vi "AlliGator Overlay Decay Fit Parameter Map in Original Image.vi"(5 "Decay Fit Parameter Map Color Scale Refnum":refnum<vi>, 7 "Image Color Scale Refnum":refnum<vi>, 8 "Error In":errorcluster, 10 "Destination Image Control Refnum":T1 caption="Source Image Refnum", 11 "AlliGator IV DVR in":refnum<data-value>) -> (0 "Error Out":errorcluster, 1 "# Overlay Pixels":i32, 3 "AlliGator IV DVR out":refnum<data-value>)   [LabVIEW 2021, in "AlliGator Decay Fit Parameter Map.lvlib"]
doc: "Overlays the Decay Fit Parameter Map on the Source Image."
uses:
  AlliGator Decay Fit Parameter Map.lvlib
  Image/Image Control Refnum.ctl
  Internal Variables/AlliGator Internal Variables v2.ctl
  <vilib>/vision/Image Controls.llb/IMAQ Image.ctl
  Internal Variables/AlliGator Gate Image Set.ctl
  Files/AlliGator FLI Dataset Type.ctl
  Files/AlliGator Data Series Type.ctl
  Dual-Channel Datasets/AlliGator Dataset Channel.ctl
  Settings/AlliGator Gate Arithmetic.ctl
  Source Image/AlliGator Displayed Image.ctl
  Image/Named ROI Description.ctl
  Phasor Graph/AlliGator Decay Metadata v3.ctl
  Decay Analysis/Decay Preprocessing/AlliGator Decay Background Subtraction Info.ctl
  Decay Analysis/Decay Preprocessing/AlliGator Baseline Subtraction Method.ctl
  Graphs/XY Graph/XY Graph Plot Shift Parameters.ctl
  Graphs/XY Graph/XY Graph Plot Shift Method.ctl
  Decay Analysis/Decay Preprocessing/AlliGator Decay Extrapolation Parameters.ctl
  Phasor/Calibration Phasor (m, phi).ctl
  Phasor/Phasor Reference Series.ctl
  Phasor/Phasor Calibration Map v2.ctl
  Phasor/Phasor (g, s).ctl
  Phasor Graph/AlliGator Raw Phasor Plot Data v4.ctl
  Phasor/Phasor Standard Deviation Options.ctl
  Phasor Plot/AlliGator Phasor Multi-Harmonic Data.ctl
  Phasor/Phasor Harmonic Data.ctl
  AlliGator Decay Fit Options & Parameters v2.ctl
  Fits/IRF(X)PSED/Decay Fit Options v2.ctl
  Fits/Decay Convolution/Decay Model.ctl
  Fits/Residual Type.ctl
  Fits/IRF(X)PSED/Fit Weights Type.ctl
  Fits/Non-linear Fitting Method v2.ctl
  Fits/Fit Calculation Method.ctl
  Fits/Non-linear Fitting Algorithm.ctl
  Decay Analysis/Decay Fit/AlliGator Decay Fit Parameter Constraints 2.ctl
  Fits/IRF(X)PSED/Decay Fit Parameters In List.ctl
  Fits/IRF(X)PSED/MLE Baseline Offset Type.ctl
  Decay Analysis/Decay Preprocessing/AlliGator Decay Preprocessing Parameters.ctl
  Fits/IRF(X)PSED/Decay Fit Parameters & Derived Quantities List v2.ctl
  AlliGator Parameter Maps Data.ctl
  Settings/AlliGator Settings List.ctl
  Palette/Limit+NaN Colors.ctl
  Globals, Variables, Constants/AlliGator Variables List.ctl
  Palette/Image Palette Information.ctl
  Image/Image Display Palette Type.ctl
  Variant/Variant to Data/Variant to Boolean.vi
  Error/Error.lvlib
  Image/Image.lvlib
  Settings/AlliGator Settings.lvlib
  Variant/Variant to Data/Variant to Data.lvlib
  <vilib>/vision/NI_Vision_Development_Module.lvlib
  Time/Time.lvlib
  Globals, Variables, Constants/AlliGator Globals, Variables & Constants.lvlib
  Palette/Palette.lvlib
  Utilities/Utilities.lvlib
  Phasor/Phasor.lvlib
  Decay Analysis/Decay Preprocessing/AlliGator Decay Preprocessing.lvlib
  Graphs/XY Graph/XY Graph Add-Ons.lvlib
  Phasor Graph/AlliGator Phasor Graph.lvlib
  Files/AlliGator Files.lvlib
  Phasor Plot/AlliGator Phasor Plot.lvlib
  Source Image/AlliGator Source Image.lvlib
  Internal Variables/AlliGator Internal Variables.lvlib
  Fits/Fits.lvlib
  Decay Analysis/Decay Fit/AlliGator Decay Fit.lvlib
  Dual-Channel Datasets/AlliGator Dual-Channel Datasets.lvlib
panel:
  out "Overlay Copy (s)":dbl
  out "Overlay Erase (s)":dbl
  out "Overlay Compute (s)":dbl
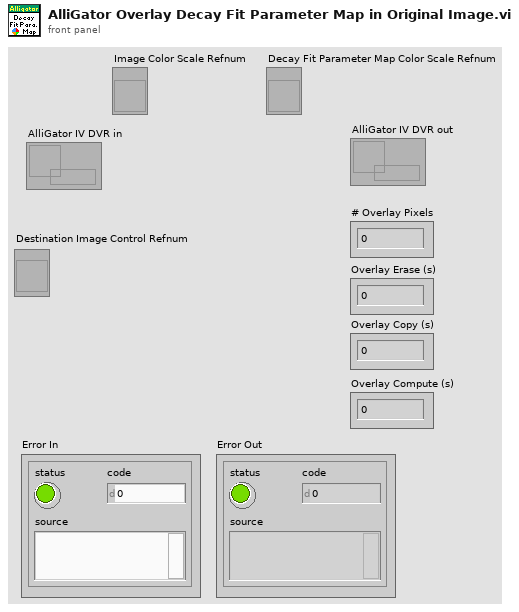
[diagram p1: front panel]
types:
  T1 = typedef "Image.lvlib/Image Control Refnum.ctl" = refnum<vi>
  T2 = typedef "Palette.lvlib/Limit+NaN Colors.ctl" = cluster{"Color Scale High Color":cluster{"Red (or Hue) value":u8, "Green (or Sat) value":u8, "Blue (or Light or Val) value":u8}, "Color Scale Low Color":cluster{"Red (or Hue) value":u8, "Green (or Sat) value":u8, "Blue (or Light or Val) value":u8}, "NaN Color":cluster{"Red (or Hue) value":u8, "Green (or Sat) value":u8, "Blue (or Light or Val) value":u8}}
  T3 = typedef "AlliGator Settings.lvlib/AlliGator Settings List.ctl" = enum16{"GUI:Visible Settings Tab", "GUI:Last Run Version", "Source Image:Use Image Histogram for Contrast", "Source Image:Low Count Pixels Rejection Options", "Source Image:High Count Pixels Rejection Options", "Source Image:Use Image Brightness", "Source Image:Blend Overlay with Image Background", "Source Image:Use Fixed ROI Diameter", "Source Image:ROI Diameter", "Source Image:ROI Center Color", "Source Image:Peak Threshold", "Source Image:Intensity Threshold", "Source Image:Image Binning Options", "Source Image:Image Smoothing Options", "Source Image:Image Histogram Active", "Source Image:Invert Binary Mask", "Source Image:Hot Pixel Removal", "Source Image:Overlay Analyzed ROI Center", "Source Image:Auto-Adjust Contrast", "Source Image:Histogram Lower Percentile", "Source Image:Histogram Upper Percentile", "Source Image:Save Source Image", "Source Image:Scale Bar Options", "Source Image:Image Resolution (Pixel Size)", "Source Image:Flatfield Correction", "Source Image:Show Dead Left Columns Correction", "Source Image:Dead Left Columns Correction", "Source Image:Image Pre-Processing Operations Order", "Source Image:Overlay ROI Median", "Source Image:Median Overlay Color", "Data Information:Gate Width", "Data Information:Nanotime Gate Separation", "Data Information:Macrotime Gate Separation", "Data Information:Gate Step", "Data Information:# Gates", "Data Information:Gate Image Exposure", "Data Information:Gate Image Integration", "Data Information:Gates to Skip", "Data Information:Gates to Keep", "Data Information:Define Gates to", "Data Information:Channel Name", "Data Information:Available Channel Names", "Data Information:Channel Arithmetic", "Data Information:Background File Subtraction", "Data Information:Background File", "Data Information:Background Scaling Factor", "Data Information:Background Pile-up Correction", "Data Information:Background Pixel Well Capacity", "Data Information:Laser Period", "Data Information:SYNC Period", "Data Information:Pile-up Correction", "Data Information:Pixel Well Capacity", "Data Information:Dataset Scaling Factor", "Fluorescence Decay_Decay Pre-Processing:Reverse Gates", "Fluorescence Decay_Decay Pre-Processing:Verbose Decay Pre-Processing", "Fluorescence Decay_Decay Pre-Processing:Use Decay Pre-Processing", "Fluorescence Decay_Decay Pre-Processing:Background Subtraction", "Fluorescence Decay_Decay Pre-Processing:Background Definition Range", "Fluorescence Decay_Decay Pre-Processing:Baseline Subtraction Method", "Fluorescence Decay_Decay Pre-Processing:Decay Pre-Processing Operations Order", "Fluorescence Decay_Decay Pre-Processing:Smoothing Parameter", "Fluorescence Decay_Decay Pre-Processing:Shift Decay", "Fluorescence Decay_Decay Pre-Processing:Decay Shift Parameters", "Fluorescence Decay_Decay Pre-Processing:Fold Decay", "Fluorescence Decay_Decay Pre-Processing:# Folds", "Fluorescence Decay_Decay Pre-Processing:1-Normalize Decay", "Fluorescence Decay_Decay Pre-Processing:[0-1]-Normalize Decay", "Fluorescence Decay_Decay Pre-Processing:Smoothen Decay", "Fluorescence Decay_Decay Pre-Processing:Extrapolate Decay", "Fluorescence Decay_Decay Pre-Processing:Use Periodicity", "Fluorescence Decay_Decay Pre-Processing:Use Cursors", "Fluorescence Decay_Decay Pre-Processing:Tail Fraction", "Fluorescence Decay_Decay Pre-Processing:Head Fraction", "Fluorescence Decay_Decay Pre-Processing:Additional Points", "Fluorescence Decay_Decay Pre-Processing:Straighten Decay", "Fluorescence Decay_Decay Pre-Processing:Constant Background", "Fluorescence Decay_Decay Pre-Processing:Pixel-Normalize Decay", "Fluorescence Decay_Advanced Analysis:Extract IRF instead of Decay", "Fluorescence Decay_Advanced Analysis:IRF Extraction Options", "Fluorescence Decay_Advanced Analysis:IRF Optimization Options", "Fluorescence Decay_Advanced Analysis:Square Pulse Options", "Fluorescence Decay_Advanced Analysis:IRF Order", "Fluorescence Decay_Advanced Analysis:IRF Time Constants", "Fluorescence Decay_Advanced Analysis:Wavelet Analysis Options", "Fluorescence Decay_Advanced Analysis:Average Lifetime Options", "Fluorescence Decay_Fit Options:Fit Options", "Fluorescence Decay_Fit Options:Use Legacy Fitting Approach", "Fluorescence Decay_Fit Options:Use Data Information Laser Period", "Fluorescence Decay_Fit Parameters:Displayed Fit Parameters", "Fluorescence Decay_Fit Parameters:Fit Parameter Constraints", "Fluorescence Decay_Fit Parameters:Export Tabulated Results", "Fluorescence Decay_Fit Parameters:MLE Baseline Offset Type", "Fluorescence Decay_Fit Parameters:MLE Baseline Offset", "Fluorescence Decay_Fit Parameters:Guess Parameter Names", "Fluorescence Decay_Fit Parameters:Guess Parameter Values", "Fluorescence Decay_Fit Parameters:Guess Parameters Options", "Fluorescence Decay_Fit Parameters:Optimal Offset Selection Criterion", "Fluorescence Decay_Styles:Show Last Decay Only", "Fluorescence Decay_Styles:Decay Graph Color Array", "Fluorescence Decay:Decay Graph Active", "Fluorescence Decay Statistics:Min Peak Value", "Fluorescence Decay Statistics:Reject Low Decay Peak Pixels", "Fluorescence Decay Statistics:Reject High Decay Peak Pixels", "Fluorescence Decay Statistics:Max Peak Value", "Time Traces:Use File Timestamp", "Time Traces:Time Step", "Time Traces:Use Intensity Correction File", "Time Traces:Intensity Correction File", "Phasor Plot:Phasor Plot Smoothing Options", "Phasor Plot:Phasor Plot Size", "Phasor Plot:Phasor Plot Graphics Options", "Phasor Plot:Cumulative Phasor Plot", "Phasor Plot:Use Phasor Brightness", "Phasor Plot:Blend Overlay with Phasor Background", "Phasor Plot:Save Phasor Plot", "Phasor Plot:Show References", "Phasor Plot:Phasor Ratio Decay Range", "Phasor Plot:Exponential Fading", "Phasor Plot:Phasor Ratio Reference Colors", "Phasor Plot:Reference Radius", "Phasor Plot:Show Color Map Vertices", "Phasor Plot:Phasor Plot Active", "Phasor Plot:Phasor Ratio Color Map Type", "Phasor Plot:Phasor Ratio Color Map", "Phasor Plot:Phasor Ratio Display Range", "Phasor Plot:Selected Image ROI(s)", "Phasor Plot:All Image ROIs", "Phasor Plot:Selected Phasor Plot ROI(s)", "Phasor Plot:All Phasor Plot ROIs", "Phasor Plot:Phasor Ratio Color-Coded Quantity", "Phasor Plot:Store Phasor Harmonics", "Phasor Plot:Draw Reference Segment", "Phasor Plot:User-Defined Quantity", "Phasor Plot:Color Scale High Color", "Phasor Plot:Color Scale Low Color", "Phasor Graph:Phasor Frequency", "Phasor Graph:Phasor Ratio Type", "Phasor Graph:Pixel-level Phasor Computation", "Phasor Graph:Save Phasor Graph", "Phasor Graph:Phasor Graph Active", "Phasor Graph:Phasor SDV Options", "Phasor Calibration:Use Backup Calibration if needed", "Phasor Graph:Define Shortest Lifetime as", "Phasor Calibration:Backup Calibration Type", "Phasor Calibration:Calibration Type", "Phasor Calibration:Calibration Lifetime", "Phasor Calibration:Calibration Map Algorithm", "Single-Exponential Phasor Locus (SEPL):Gate Parameters", "Single-Exponential Phasor Locus (SEPL):User-defined Gate", "Single-Exponential Phasor Locus (SEPL):User-defined IRF", "Single-Exponential Phasor Locus (SEPL):Phasor Parameters", "Single-Exponential Phasor Locus (SEPL):Decay & IRF Parameters", "Single-Exponential Phasor Locus (SEPL):Display Parameters", "Lifetime Analysis:Decay Analysis Parameters", "Lifetime Analysis:Lifetime Map Active", "Plugins:Python Settings", "Miscellaneous:Verbose Mode", "Miscellaneous:Beep after Script", "Miscellaneous:Saved Image File Format", "Miscellaneous:Exported Gate Image Settings", "Miscellaneous:Include Loading in Timing", "Miscellaneous:Verbose Settings Mode", "Miscellaneous:Histogram Options", "Miscellaneous:Beep on Error", "Miscellaneous:# Logical Processors Used", "Miscellaneous:ROI Description Max Characters", "Miscellaneous:Verbose Error Mode", "Miscellaneous:Transparent Mask Color"}
  T4 = cluster{"Red (or Hue) value":u8, "Green (or Sat) value":u8, "Blue (or Light or Val) value":u8}
  T5 = typedef "IMAQ Image.ctl" = refnum<image>
  T6 = typedef "AlliGator Globals, Variables & Constants.lvlib/AlliGator Variables List.ctl" = enum16{"---- GUI ----", "GUI:Initialization Status", "GUI:State Indicators Refnum", "GUI:Original AlliGator Menu Items", "GUI:Current Action Loop State", "GUI:Script in progress", "GUI:Playback", "GUI:Loop Playback", "GUI:Search ROI Used", "GUI:Search ROI", "Decay Graph Max Legend Size", "Intensity Graph Max Legend Size", "Decay Statistics Graph Max Legend Size", "Phasor Graph Max Legend Size", "Phasor Ratio Graph Max Legend Size", "Lifetime Graph Max Legend Size", "---- Files ----", "Files:Export Dataset Frames as Individual Files", "Files:Show Batch Export Help Balloons", "Files:Frames in Dataset", "Files:ptu File Frame Start Indices", "Files:Current Frame in Dataset", "Files:Current Frame Timestamp", "Files:Dataset Loaded", "Files:Dataset Metadata", "Files:Dataset Channel", "Files:Dataset Data Description", "Files:Background Dataset Metadata", "Files:Background Dataset Channel", "Files:Background Dataset Data Description", "Files:Background File Subtraction", "Files:Background File Path", "Files:Background File Pile-up Correction", "Files:Background File Pixel Well Capacity", "Files:Background File Scaling Factor", "Files:Current Dataset Load Settings", "Files:Dataset Path", "Files:ICCD-specific Information", "Files:Macrotime Gate Separation", "------ Python Plugins ------", "Python Plugins:Information", "Python Plugins:Python Session", "Python Plugins:Valid Python Session?", "---- Source Image ----", "Source Image:ROIs", "Source Image:Current ROI", "Source Image:ROI Event Refnum", "X_Source Image:Display Range", "X_Source Image:Palette Information", "X_Source Image:Type of Displayed Image", "X_Time Gate Slider", "Source Image:Palette List", "Source Image:Scale", "Source Image:ROI Overlay Color", "Source Image:Overlay to Erase", "Source Image:Is Displayed Image Accumulated", "Source Image:White Light Image Modified", "Source Image:Mask Image Modified", "---- Image Profile Window ----", "Image Profile:Window Event Refnum", "Image Profile:IntensityType", "Image Profile:Intensity Average Type", "Image Profile:Intensity-weighted SDV", "Image Profile:Box Profile Type", "Image Profile:Window Open", "Image Profile:Plotted Fit Parameter", "------ Phasor Graph -------", "Phasor Graph:Show Line", "---- Phasor Plot ---", "Phasor Plot:Parameters Changed", "Phasor Plot:FLI Dataset Modified since last Calculation", "Phasor Harmonics Data", "Selected Phasor Harmonics", "Phasor Harmonic Manager Event Refnum", "Phasor Plot:ROIs", "Phasor Plot:Current ROI", "Phasor Plot:ROI Event Refnum", "Phasor Plot:Image Reference Points", "Phasor Plot:Computed", "Phasor Plot:Palette Information", "Phasor Plot:Palette List", "Phasor Plot:Phasor Ratio Palette Information", "Phasor Plot:Phasor Ratio Palette List", "Phasor Plot:Image Scale", "Phasor Plot:Image Overlay to Erase", "Phasor Plot:Image Elements to Update", "Phasor Plot:Current Calculation Parameters", "Phasor Plot:Current Calibration Options", "Phasor Plot:Reset Cumulated Phasor Plot", "Phasor Plot:Reference 1", "Phasor Plot:Lifetime Reference 1", "Phasor Plot:Reference 1 Frequency", "Phasor Plot:Reference 2", "Phasor Plot:Lifetime Reference 2", "Phasor Plot:Reference 2 Frequency", "---- Decay Analysis ----", "Number of Selected Decays to Fit", "LS Fit Results", "LAR Fit Results", "BS Fit Results", "Last Decay Max - Min", "Best Fit Parameters", "Best Fit Parameter Names", "Actual Size X", "Actual Size Y", "Binning X", "Binning Y", "Actual # Gates", "Dataset Number", "Gates to...", "Gates Skipped", "Gates to keep", "Gate Step", "Gate Separation", "Reversed Gates", "Pile-up Correction", "Pixel Well Capacity", "Background Subtracted", "Background Subtraction Method", "Background Definition Range", "Background File (deprecated)", "Number of Dataset Accumulated", "Array of Accumulated Dataset Paths", "Do Averaged Datasets", "Destination File Path", "Process Plot Target", "Use 1/D as Phasor Frequency", "---- Decay Fit Parameter Map -----", "Decay Fit Parameter Map:Palette Information", "Decay Fit Parameter Map:Palette List", "Decay Fit Parameter Map:X Resolution", "Decay Fit Parameter Map:Y Resolution", "---- Parameter Map ----", "Parameter Map:Palette Information", "Parameter Map:Palette List", "------- Local Decay Window ---------", "Local Decay Graph Window:Event Refnum", "Local Decay Graph Window:Use normalized IRF for convolution", "----- Miscellaneous ----", "Misc:Skippable Dialog Windows Status"}
  T7 = typedef "Palette.lvlib/Image Palette Information.ctl" = cluster{"Palette Name [# Colors,int?,inv?]":string, "Palette Type":T8, "Palette Colors":u32[], "Interpolate?":bool}
  T8 = typedef "Image.lvlib/Image Display Palette Type.ctl" = u32
  T9 = typedef "AlliGator Internal Variables.lvlib/AlliGator Internal Variables v2.ctl" = cluster{"Displayed Image":T5, "White Light Image":T5, "Mask Image":T5, "ROI Mask Image":T5, "Current Dataset Images 1":T10, "Background Dataset Images 1":T10, "Current Dataset Images 2":T10, "Background Dataset Images 2":T10, "Current Dataset Arithmetic Images":T10, "Accumulated Dataset Images 1":T10, "Accumulated Dataset Images 2":T10, "Accumulated Dataset Arithmetic Images":T10, "Phasor Plot Image":T5, "Decay Fit Parameter Map Image":T5, "Parameter Map Image":T5, "Single Data Point Path":path, "White Light Image Path":path, "Mask Image Path":path, "Time-Series Folder":path, "[Time-Series Paths]":path[], "Current Dataset":i32, "Single Dataset Type":T11, "Current Folder":string, "AlliGator Data Series Type":T12, "# Datasets":i32, "Dual-Channel Dataset":bool, "Selected Channel Name":string, "Dataset Channel":T13, "Channel Arithmetic":T14, "Dual-Channel Background Dataset":bool, "Background Channel":T13, "Dual-Channel Accumulated Dataset":bool, "Start Time":dbl, "[Time-Series Timestamps]":dbl[], "[Intensity Corrections]":dbl[], "Time Series Script":bool, "Type of Displayed Image":T15, "Gate Image Slide":u16, "# Gates":i32, "ROIs":T16[], "ROI Decay":cluster{"t Array":dbl[], "I Array":dbl[]}, "Valid Decay":bool, "Decay  Metadata":T18, "Reference Decay Plot Name":string, "Reference Decay":cluster{"t Array":dbl[], "I Array":dbl[]}, "Decay Shift Plot":cluster{"Time Stamps":dbl[], "Decay Shifts":dbl[]}, "[Decays Max Values]":sgl[], "[Decays Min Values]":sgl[], "Calibration Phasor":T24, "Calibration Phasor Series":T25, "Phasor Calibration Map":T26, "Calibration Map MD5 Digest":string, "Last Raw Phasor":T27, "Last Calibrated Phasor":T27, "Last Calibrated Phasor SDV":T27, "Phasor Graph:Phasor Plot":cluster{"g Array":dbl[], "s Array":dbl[]}, "Phasor Graph:Phasor SDV Plot":cluster{"g Array":dbl[], "s Array":dbl[]}, "[Phasor Graph:Raw Phasor Plots]":T28[], "Phasor Plot locked to Ref 1":i32, "[Phasor Plot(s) locked to Ref 1]":i32[], "[Phasor Plot(s) locked to Ref 2]":i32[], "[Pixel Phasors]":T27[], "[[Sum Image]]":dbl[][], "[[CSG Phasors]]":csg[][], "[[Valid Pixel?]]":bool[][], "I/m/phi Dataset":cluster{"I/m/phi Dataset?":bool, "Base Frequency":dbl[unit], "Harmonic Orders":u8[]}, "Multi Phasor Plot Data":T30, "Decay Fit Options & Parameters":T32, "Fit Options: Decay Preprocessing Parameters":T43, "Fit Options: Reference Decay":cluster{"t Array":dbl[], "I Array":dbl[]}, "Is Full Image Parameters Map":bool, "Is Single-Pixels Parameters Map":bool, "NLSF Parameters Map X Resolution":i32, "NLSF Parameters Map Y Resolution":i32, "[Single Decay Fit Parameters]":dbl[], "Fit Model":T34, "[[Multiple Decays Fit Parameters]]":dbl[][], "[[Multiple Decays Fit Parameter SDVs]]":dbl[][], "[[IRFs]]":dbl[][], "IRF Array Time Axis":dbl[], "Decay Array Time Axis":dbl[], "[Decay Fit Parameter Names]":T44[], "[[Phasor Ratios]]":dbl[][], "[[Average Lifetimes]]":dbl[][], "Amplitude Weighted Average Lifetime":bool, "[Decay Sum]":dbl[], "[Map Set Names]":string[], "[Parameter Maps]":T45[], "[[User-defined Quantities]]":dbl[][], "User-defined Quantity":string}
  T10 = typedef "AlliGator Internal Variables.lvlib/AlliGator Gate Image Set.ctl" = cluster{"SGL Image Max":T5, "SGL Image Sum":T5, "SGL Gate Images":T5[], "SGL Image Min":T5}
  T11 = typedef "AlliGator Files.lvlib/AlliGator FLI Dataset Type.ctl" = enum16{"HDF5 FLI Dataset", "Gate Image Folder", ".sdt FLI Dataset (Becker & Hickl)", ".ptu FLI Dataset (PicoQuant)", "SS1 FLI Dataset", "SS2 FLI Dataset", "I/m/phi Dataset", ".bin FLI Dataset (PicoQuant Binned)", ".bin FLI Dataset (Piccolo Binned)", ".mat FLI Dataset"}
  T12 = typedef "AlliGator Files.lvlib/AlliGator Data Series Type.ctl" = enum16{"Not a Supported Series", "Gate Images Folder Series", "SwissSPAD 2 Dataset Series", "B&H FLI Dataset Series", "PicoQuant PTU FLI Dataset Series", "PicoQuant BIN FLI Dataset Series", "Piccolo hist BIN FLI Dataset Series", "HDF5 FLI Dataset Series"}
  T13 = typedef "AlliGator Dual-Channel Datasets.lvlib/AlliGator Dataset Channel.ctl" = enum16{"G2", "INT"}
  T14 = typedef "AlliGator Settings.lvlib/AlliGator Gate Arithmetic.ctl" = enum16{"None", "INT-G2", "G2/INT*<INT>", "(1 - G2/INT)*<INT>"}
  T15 = typedef "AlliGator Source Image.lvlib/AlliGator Displayed Image.ctl" = enum16{"Single Gate", "Sum of All Gates", "Max of All Gates", "Min of All Gates", "-", "White Ligth Image", "Mask Image"}
  T16 = typedef "Image.lvlib/Named ROI Description.ctl" = cluster{"ROI Descriptor":T17, "ROI Name":string, "Overlay Color":u32}
  T17 = typedef "ROI Descriptor" = cluster{"Global Rectangle":i32[], "Contours":cluster{"ID":enum32{"External", "Internal"}, "Type":u32, "Coordinates":i32[]}[]}
  T18 = typedef "AlliGator Phasor Graph.lvlib/AlliGator Decay Metadata v3.ctl" = cluster{"ROI Descriptor":T17, "ROI Center":cluster{"X":i32, "Y":i32}, "Decay Background Subtraction Info":T19, "Decay Reverted":bool, "Decay Smoothened":bool, "Decay Straightened":bool, "Fitted Tau (Decay Straightening)":dbl, "Decay Shift Parameters":T21, "Decay Shifted":bool, "Decay Extrapolated":bool, "Decay Extrapolation Parameters":T23, "Decay Normalized":bool, "Fold Decay":bool, "# Folds":u32}
  T19 = typedef "AlliGator Decay Preprocessing.lvlib/AlliGator Decay Background Subtraction Info.ctl" = cluster{"Laser Period":dbl[unit], "Gate Duration":dbl[unit], "Baseline Subtraction Method":T20, "Background Definition Range":cluster{"Min Gate":dbl[unit], "Max Gate":dbl[unit]}, "Total Intensity w/o Bkgd Subtraction":dbl, "Bkgd-subtracted Intensity (exp)":dbl, "# Data Points":i32, "Background/Gate":dbl, "Fitted Lifetime":dbl[unit], "Bkgd-subtracted Intensity (theo)":dbl}
  T20 = typedef "AlliGator Decay Preprocessing.lvlib/AlliGator Baseline Subtraction Method.ctl" = enum16{"Mean", "Min", "Square Gated Single-Exponential", "File", "Constant"}
  T21 = typedef "XY Graph Add-Ons.lvlib/XY Graph Plot Shift Parameters.ctl" = cluster{"Type":T22, "Shift":dbl[unit], "Threshold":dbl, "Rotate":bool}
  T22 = typedef "XY Graph Add-Ons.lvlib/XY Graph Plot Shift Method.ctl" = enum16{"Default", "CFD", "Threshold", "Cross-Correlation"}
  T23 = typedef "AlliGator Decay Preprocessing.lvlib/AlliGator Decay Extrapolation Parameters.ctl" = cluster{"Additional Points":u32, "Head Fraction":dbl, "Fitted Tau":dbl, "Use Periodicity":bool, "Use Cursors":bool, "Tail Fraction":dbl}
  T24 = typedef "Phasor.lvlib/Calibration Phasor (m, phi).ctl" = cluster{"m":dbl, "phi":dbl, "Phasor Frequency":dbl[unit], "Reference Lifetime":dbl[unit]}
  T25 = typedef "Phasor.lvlib/Phasor Reference Series.ctl" = cluster{"m Array":dbl[], "phi Array":dbl[], "Phasor Frequency":dbl[unit], "Calibration Lifetime":dbl[unit]}
  T26 = typedef "Phasor.lvlib/Phasor Calibration Map v2.ctl" = cluster{"Phasor Frequency":dbl[unit], "Calibration Lifetime":dbl[unit], "ROI Centers":cluster{"X":i32, "Y":i32}[], "ROI Descriptors":T17[], "Map Resolution X":i32, "Map Resolution Y":i32, "z Array":cdb[]}
  T27 = typedef "Phasor.lvlib/Phasor (g, s).ctl" = cluster{"g":dbl, "s":dbl}
  T28 = typedef "AlliGator Phasor Graph.lvlib/AlliGator Raw Phasor Plot Data v4.ctl" = cluster{"Phasor Plot Name":string, "Raw Phasor Plot":T27[], "Phasor Frequency":dbl[unit], "[Decay Metadata]":T18[], "Raw Phasor Plot SDV":T27[], "Phasor SDV Options":T29, "[Calibration Phasor]":T24[]}
  T29 = typedef "Phasor.lvlib/Phasor Standard Deviation Options.ctl" = cluster{"Compute Estimated SDV":bool, "# Replicas":u32, "Use Estimated Average Phasor":bool}
  T30 = typedef "AlliGator Phasor Plot.lvlib/AlliGator Phasor Multi-Harmonic Data.ctl" = cluster{"Base Frequency":dbl[unit], "# Harmonics":u8, "Harmonic Orders":u8[], "Phasor Plot Settings Checksum":u64, "Phasor Harmonic Data Array":T31[]}
  T31 = typedef "Phasor.lvlib/Phasor Harmonic Data.ctl" = cluster{"Phasor Harmonic Name":string, "Phasor Plot Settings Checksum":u64, "Phasor Frequency":dbl[unit], "Base Frequency":dbl[unit], "Harmonic Order":u8, "Phasor Plot Parameters":string, "Phasor Array [[CSG]]":csg[][], "Dataset File Path":path}
  T32 = typedef "AlliGator Decay Fit Parameter Map.lvlib/AlliGator Decay Fit Options & Parameters v2.ctl" = cluster{"SYNC Period":dbl[unit], "Fit Options":T33, "Fit Parameter Constraints":T40[], "MLE Baseline Offset":dbl, "MLE Baseline Offset Type":T42}
  T33 = typedef "Fits.lvlib/Decay Fit Options v2.ctl" = cluster{"Show Fit Residuals":bool, "Fit Model":T34, "Residual Type":T35, "Max Decay Percentile":dbl, "Min Decay Percentile":dbl, "Show Full Decay":bool, "Weights":T36, "Fitting Method":T37, "Compute Parameter Uncertainties":bool, "Periodic Boundaries":bool, "Model Calculation":T38, "Period":dbl[unit], "Termination Criteria":cluster{"Max Iterations":i32, "Max Function Calls":i32, "Max Time":dbl[unit], "Function Tolerance":dbl, "Parameter Tolerance":dbl, "Gradient Tolerance":dbl, "Min Lambda":dbl, "Max Lambda":dbl, "Initial Tick Count":u32}, "Offset Resolution":dbl[unit], "Use Local IRF":bool, "Fitting Algorithm":T39}
  T34 = typedef "Fits.lvlib/Decay Model.ctl" = enum16{"1-Exponential", "2-Exponentials"}
  T35 = typedef "Fits.lvlib/Residual Type.ctl" = enum16{"Standard", "Normalized", "Reduced"}
  T36 = typedef "Fits.lvlib/Fit Weights Type.ctl" = enum16{"Unweighted", "1/Variance", "Best of All"}
  T37 = typedef "Fits.lvlib/Non-linear Fitting Method v2.ctl" = enum16{"Least Square", "Least Absolute Residual", "Bisquare", "MLE", "-", "Best of All"}
  T38 = typedef "Fits.lvlib/Fit Calculation Method.ctl" = enum16{"Simulation", "Convolution", "Integration"}
  T39 = typedef "Fits.lvlib/Non-linear Fitting Algorithm.ctl" = enum16{"Levenberg-Marquardt", "Trust-Region Dogleg"}
  T40 = typedef "AlliGator Decay Fit.lvlib/AlliGator Decay Fit Parameter Constraints 2.ctl" = cluster{"Fit Parameter":T41, "Min Value":dbl, "Max Value":dbl, "Global":bool, "Used":bool}
  T41 = typedef "Fits.lvlib/Decay Fit Parameters In List.ctl" = enum16{"Offset", "Baseline", "A_1", "tau_1", "A_2", "tau_2"}
  T42 = typedef "Fits.lvlib/MLE Baseline Offset Type.ctl" = enum32{"Absolute", "Percentage"}
  T43 = typedef "AlliGator Decay Preprocessing.lvlib/AlliGator Decay Preprocessing Parameters.ctl" = cluster{"Background Subtraction":bool, "Straighten Decay":bool, "Reverse Gates":bool, "1-Normalized Decay":bool, "Smoothen Decay":bool, "Smoothing Parameter":dbl, "Shift Decay":bool, "Decay Shift Parameters":T21, "Extrapolate Decay":bool, "Additional Points":u32, "Head Fraction":dbl, "Pixel-Normalize Decay":bool, "Use Periodicity":bool, "Use Cursors":bool, "Tail Fraction":dbl, "Use Decay Pre-Processing":bool, "Fold Decay":bool, "# Folds":u32, "[0-1]-Normalized Decay":bool}
  T44 = typedef "Fits.lvlib/Decay Fit Parameters & Derived Quantities List v2.ctl" = enum16{"Offset", "Baseline", "A_1", "tau_1", "A_2", "tau_2", "<tau>_a", "f1_a", "f2_a", "<tau>_i", "f1_i", "f2_i", "-", "R^2", "Chi^2"}
  T45 = typedef "AlliGator Decay Fit Parameter Map.lvlib/AlliGator Parameter Maps Data.ctl" = cluster{"Map Set Name":string, "[Parameter Names]":string[], "[[Parameters]]":dbl[][], "[[Parameter SDVs]]":dbl[][], "Decay Array Time Axis":dbl[], "[[IRFs]]":dbl[][], "IRF Array Time Axis":dbl[]}
  T46 = cluster{"Red (or Hue) value":u8, "Green (or Sat) value":u8, "Blue (or Light or Val) value":u8}[]
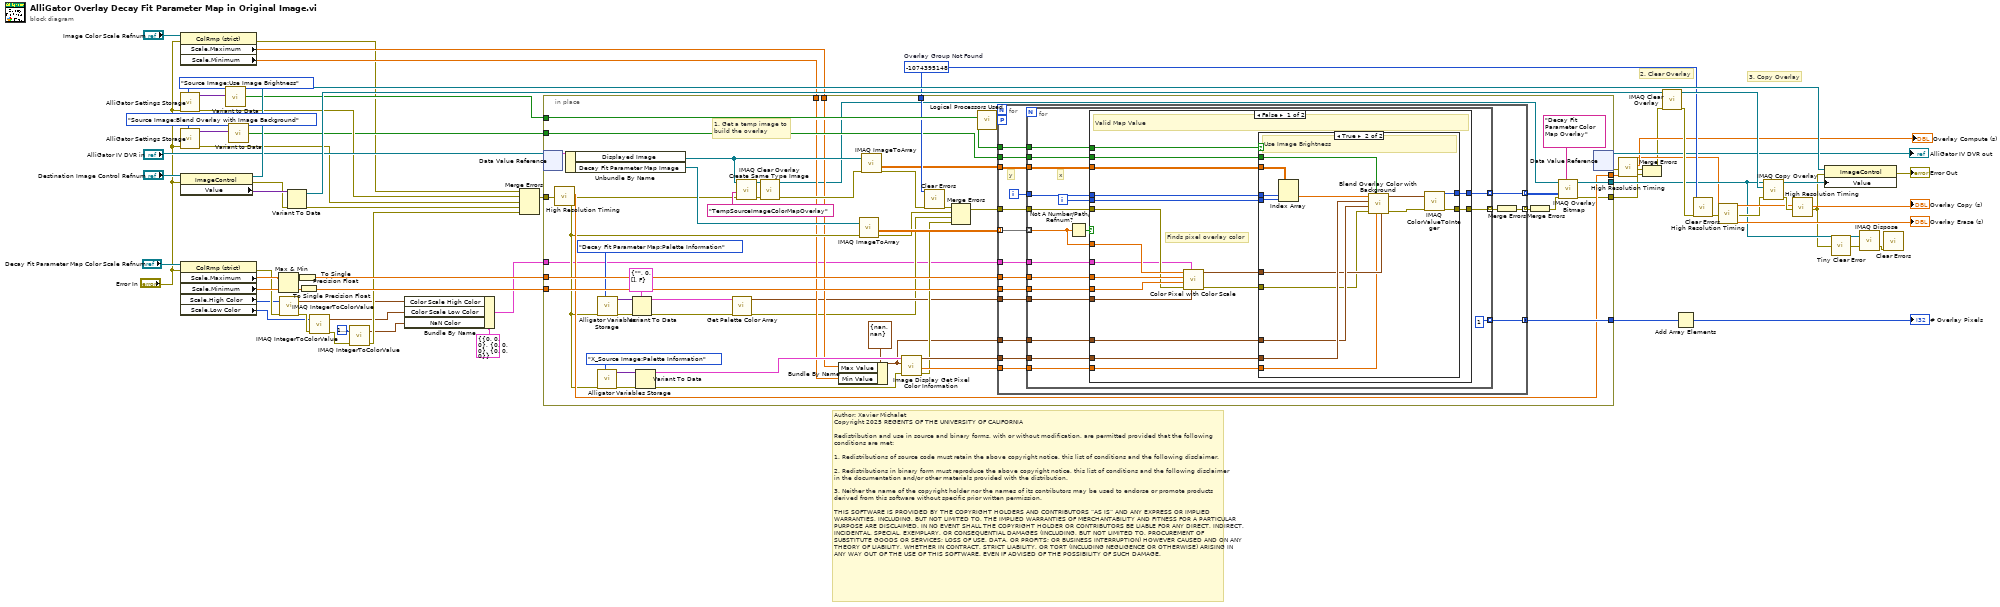
[diagram p0: block diagram]
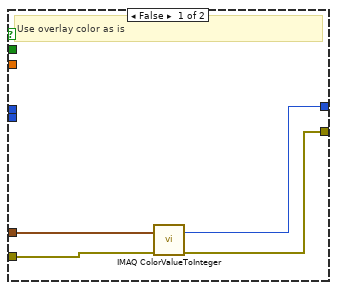
[diagram p2: hidden frame]
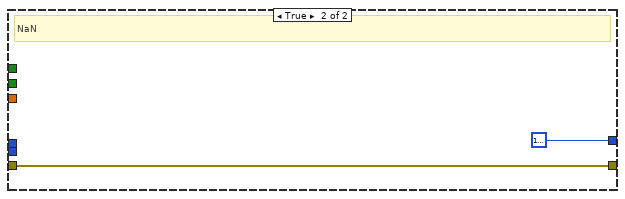
[diagram p3: hidden frame]
diagram:
  w51 = -1074395148  # Overlay Group Not Found
  # "Author: Xavier Michalet\nCopyright 2025 REGENTS OF THE UNIVERSITY OF CALIFORNIA\n\nRedistribution and use in source and binary forms, with or without modification, are permitted provided that the following conditions are met:\n\n1. Redistributions of source code must retain the above copyright notice, this list of conditions and the following disclaimer.\n\n2. Redistributions in binary form must reproduce the above copyright notice, this list of conditions and the following disclaimer in the documentation and/or other materials provided with the distribution.\n\n3. Neither the name of the copyright holder nor the names of its contributors may be used to endorse or promote products derived from this software without specific prior written permission.\n\nTHIS SOFTWARE IS PROVIDED BY THE COPYRIGHT HOLDERS AND CONTRIBUTORS “AS IS” AND ANY EXPRESS OR IMPLIED WARRANTIES, INCLUDING, BUT NOT LIMITED TO, THE IMPLIED WARRANTIES OF MERCHANTABILITY AND FITNESS FOR A PARTICULAR PURPOSE ARE DISCLAIMED. IN NO EVENT SHALL THE COPYRIGHT HOLDER OR CONTRIBUTORS BE LIABLE FOR ANY DIRECT, INDIRECT, INCIDENTAL, SPECIAL, EXEMPLARY, OR CONSEQUENTIAL DAMAGES (INCLUDING, BUT NOT LIMITED TO, PROCUREMENT OF SUBSTITUTE GOODS OR SERVICES; LOSS OF USE, DATA, OR PROFITS; OR BUSINESS INTERRUPTION) HOWEVER CAUSED AND ON ANY THEORY OF LIABILITY, WHETHER IN CONTRACT, STRICT LIABILITY, OR TORT (INCLUDING NEGLIGENCE OR OTHERWISE) ARISING IN ANY WAY OUT OF THE USE OF THIS SOFTWARE, EVEN IF ADVISED OF THE POSSIBILITY OF SUCH DAMAGE."
  # "3. Copy Overlay"
  # "2. Clear Overlay"
  n1 = property class="ColRmp (strict)"(reference="Image Color Scale Refnum", error in="Error In") -> (error out=w12:errorcluster, "Scale.Maximum"=w15:dbl, "Scale.Minimum"=w14:dbl)  [unwired: 1 out]
  n2 = call "AlliGator Settings Storage.vi"("AlliGator Settings List"=AlliGator_Settings_List."Source Image:Use Image Brightness", "Error In"="Error In") -> ("Error Out"=w36:errorcluster, "Variant Data out"=w56:variant)  [unwired: 8 in]
  n3 = call "AlliGator Settings Storage.vi"("AlliGator Settings List"=AlliGator_Settings_List."Source Image:Blend Overlay with Image Background", "Error In"="Error In") -> ("Error Out"=w23:errorcluster, "Variant Data out"=w26:variant)  [unwired: 8 in]
  n4 = property class="ImageControl"(reference="Destination Image Control Refnum", error in="Error In") -> (reference out=w61:T1, error out=w63:errorcluster, "Value"=w64:variant)
  n5 = property class="ColRmp (strict)"(reference="Decay Fit Parameter Map Color Scale Refnum", error in="Error In") -> (error out=w11:errorcluster, "Scale.Maximum"=w33:dbl, "Scale.Minimum"=w32:dbl, "Scale.High Color"=w10:u32, "Scale.Low Color"=w9:u32)  [unwired: 1 out]
  n6 = call-poly "Variant to Data.vi"("Variant"=w56) -> ("Value"=w53:bool)  [unwired: 8 in]
  n7 = call-poly "Variant to Data.vi"("Variant"=w26) -> ("Value"=w22:bool)  [unwired: 8 in]
  n8 = Max & Min(x=w33, y=w32) -> (max(x,y)=w31:dbl, min(x,y)=w30:dbl)
  n9 = call "IMAQ IntegerToColorValue"("error in (no error)"=w11, "U32 value"=w10) -> ("error out"=w13:errorcluster, "Color Value"=w4:T4)  [unwired: 3 in, 2 out]
  n10 = Variant To Data(error in=w63, Variant=w64) -> (data=w55:T5, error out=w54:errorcluster)  [unwired: 1 in]
  n11 = To Single Precision Float(number=w31) -> (single precision float=w29:sgl)
  n12 = To Single Precision Float(number=w30) -> (single precision float=w28:sgl)
  n13 = call "IMAQ IntegerToColorValue"("error in (no error)"=w13, "U32 value"=w9) -> ("error out"=w7:errorcluster, "Color Value"=w3:T4)  [unwired: 3 in, 2 out]
  n14 = call "IMAQ IntegerToColorValue"("error in (no error)"=w7, "U32 value"=u32 16777216) -> ("error out"=w6:errorcluster, "Color Value"=w2:T4)  [unwired: 3 in, 2 out]
  n15 = Bundle By Name(cluster=T2 {"Color Scale High Color"={"Red (or Hue) value"=0, "Green (or Sat) value"=0, "Blue (or Light or Val) value"=0}, "Color Scale Low Color"={"Red (or Hue) value"=0, "Green (or Sat) value"=0, "Blue (or Light or Val) value"=0}, "NaN Color"={"Red (or Hue) value"=0, "Green (or Sat) value"=0, "Blue (or Light or Val) value"=0}} ("Limit Colors"), "Color Scale High Color"=w4, "Color Scale Low Color"=w3, "NaN Color"=w2) -> (w1:T2)
  n16 = Merge Errors(w12, w36, w23, w54, w6) -> (w37:errorcluster)
  n17 = in-place {
    in-place-border: [w116] -> w60
    in-place-border: [w115] -> w41
    in-place-border: w37 -> [w114]
    in-place-border: w53 -> [w113]
    in-place-border: w51 -> [w112]
    in-place-border: w29 -> [w110]
    in-place-border: w28 -> [w109]
    in-place-border: w22 -> [w93]
    in-place-border: [w92] -> w20
    in-place-border: [w78] -> w16
    in-place-border: w15 -> [w73]
    in-place-border: w14 -> [w72]
    in-place-border: w1 -> [w66]
    # "1. Get a temp image to\nbuild the overlay"
    n18 = in-place-dvr #1("AlliGator IV DVR in") -> (w111:T9)  [unwired: 1 out]
    n19 = call "High Resolution Timing.vi"("Error In"=w114) -> ("elapsed (relative) seconds"=w92:dbl, "Error Out"=w86:errorcluster)  [unwired: 16 in, 1 out]
    n20 = Unbundle By Name(w111) -> ("Displayed Image"=w94:T5, "Decay Fit Parameter Map Image"=w98:T5)
    n21 = call "Alligator Variables Storage.vi"("AlliGator Variable"=AlliGator_Variables_List."X_Source Image:Palette Information" ("Alligator Variable"), "Error In"=w86) -> ("Error Out"=w89:errorcluster, "Data out"=w90:variant)  [unwired: 7 in, 1 out]
    n22 = call "Alligator Variables Storage.vi"("AlliGator Variable"=AlliGator_Variables_List."Decay Fit Parameter Map:Palette Information" ("Alligator Variable"), "Error In"=w86) -> ("Error Out"=w101:errorcluster, "Data out"=w102:variant)  [unwired: 7 in, 1 out]
    n23 = Variant To Data(error in=w101, type=T7 {"Palette Name [# Colors,int?,inv?]"="", "Palette Type"=0, "Palette Colors"=[], "Interpolate?"=FALSE} ("Image Display Palette Information"), Variant=w102) -> (data=w99:T7, error out=w68:errorcluster)
    n24 = Variant To Data(error in=w89, Variant=w90) -> (data=w91:T7, error out=w83:errorcluster)  [unwired: 1 in]
    n25 = call "Get Palette Color Array.vi"("error in (no error)"=w68, "Image Display Palette Information"=w99) -> ("error out"=w67:errorcluster, "1D Color value array"=w70:T46)  [unwired: 8 in]
    n26 = call "Create Same Type Image.vi"("error in (no error)"=w86, "Name in"="TempSourceImageColorMapOverlay", "Image Src"=w94) -> ("error out"=w106:errorcluster, "Image Dst"=w107:T5)  [unwired: 6 in, 1 out]
    n27 = call "IMAQ Clear Overlay"("error in (no error)"=w106, "Image"=w107) -> ("error out"=w96:errorcluster, "Image Out"=w69:T5)  [unwired: 8 in]
    n28 = Bundle By Name(cluster=cluster{"Min Value":sgl, "Max Value":sgl} {"Min Value"=nan, "Max Value"=nan} ("Image Display Range"), "Max Value"=w73, "Min Value"=w72) -> (w71:cluster{"Min Value":sgl, "Max Value":sgl})
    n29 = call "IMAQ ImageToArray"("error in (no error)"=w86, "Image"=w98) -> ("Image Pixels (Float)"=w97:sgl[][], "error out"=w81:errorcluster)  [unwired: 2 in, 3 out]
    n30 = call "IMAQ ImageToArray"("error in (no error)"=w96, "Image"=w94) -> ("Image Pixels (Float)"=w79:sgl[][], "error out"=w95:errorcluster)  [unwired: 2 in, 3 out]
    n31 = call "Image Display Get Pixel Color Information.vi"("Error In"=w83, "Image Display Range"=w71, "Image Display Palette Information"=w91) -> ("Error Out"=w80:errorcluster, "Image Scale Factor (256 colors)"=w84:sgl, "1D Color Array"=w85:cluster{"Red":u8, "Green":u8, "Blue":u8}[])  [unwired: 5 in, 1 out]
    n32 = call <vilib>:"Clear Errors.vi"("error in (no error)"=w95, "specific error code to clear (0: all)"=w112) -> ("error out"=w105:errorcluster)  [unwired: 4 in, 1 out]
    n33 = Merge Errors(w105, w81, w67, w80) -> (w82:errorcluster)
    n34 = call "Logical Processors Used.vi"() -> ("# Logical Processor Used"=w77:i32)  [unwired: 6 in]
    n35 = for {
      tunnel: w113 -> [w130]
      tunnel: w82 -> [w132]
      tunnel: [w131] -> w116 mode=concatenating
      tunnel: w110 -> [w129]
      tunnel: w109 -> [w128]
      tunnel: w97 -> [w127] mode=indexing
      tunnel: w79 -> [w126]
      workers-P: w77 -> [_]
      tunnel: w93 -> [w125]
      tunnel: w85 -> [w124]
      tunnel: w84 -> [w123]
      tunnel: [w122] -> w75 mode=indexing
      tunnel: [w120] -> w76 mode=indexing
      tunnel: w71 -> [w119]
      tunnel: w70 -> [w118]
      tunnel: w66 -> [w117]
      i -> [w133]
      # "y"
      n36 = for {
        tunnel: w133 -> [w148]
        tunnel: w130 -> [w149]
        tunnel: w132 -> [w151]
        tunnel: [1] -> w131 mode=indexing
        tunnel: w129 -> [w146]
        tunnel: w128 -> [w145]
        tunnel: w127 -> [w142] mode=indexing
        tunnel: w126 -> [w143]
        tunnel: w125 -> [w141]
        tunnel: w124 -> [w140]
        tunnel: w123 -> [w139]
        tunnel: [w138] -> w122 mode=indexing
        tunnel: [w137] -> w121 mode=indexing
        tunnel: w119 -> [w136]
        tunnel: w118 -> [w135]
        tunnel: w117 -> [w134]
        i -> [w147]
        # "x"
        n37 = Not A Number/Path/Refnum?(number/path/refnum=w142) -> (NaN/Path/Refnum?=w144:bool)
        n38 = case shown="False" w144 {
          tunnel: [w160 w189] -> w137
          tunnel: w149 -> [w169 _]
          tunnel: w148 -> [w168 _]
          tunnel: w147 -> [w167 _]
          tunnel: w151 -> [w155 w189]
          tunnel: w146 -> [w157 _]
          tunnel: w145 -> [w156 _]
          tunnel: w142 -> [w158 _]
          tunnel: w143 -> [w165 _]
          tunnel: w141 -> [w164 _]
          tunnel: w140 -> [w163 _]
          tunnel: w139 -> [w162 _]
          tunnel: [w161 u32 16777216] -> w138
          tunnel: w136 -> [w159 _]
          tunnel: w135 -> [w153 _]
          tunnel: w134 -> [w152 _]
          frame False {
            # "Finds pixel overlay color"
            # "Valid Map Value"
            n39 = call "Color Pixel with Color Scale.vi"("Color Scale 1D Color Array"=w153, "Limit+NaN Colors"=w152, "Error In"=w155, "Color Scale Min Value"=w156, "Color Scale Max Value"=w157, "Pixel Value"=w158) -> ("Error Out"=w154:errorcluster, "Pixel Color"=w166:T4)  [unwired: 4 in]
            n40 = case shown="True" w169 {
              tunnel: w168 -> [_ w184]
              tunnel: w167 -> [_ w183]
              tunnel: [w172 w187] -> w161
              tunnel: [w171 w186] -> w160
              tunnel: w166 -> [w173 w176]
              tunnel: w165 -> [_ w185]
              tunnel: w164 -> [_ w179]
              tunnel: w163 -> [_ w178]
              tunnel: w162 -> [_ w175]
              tunnel: w159 -> [_ w177]
              tunnel: w154 -> [w170 w174]
              frame False {
                # "Use overlay color as is"
                n41 = call "IMAQ ColorValueToInteger"("error in (no error)"=w170, "Color Value"=w173) -> ("error out"=w171:errorcluster, "U32 value"=w172:u32)  [unwired: 3 in, 2 out]
              }
              frame True {
                # "Use Image Brightness"
                n42 = Index Array(array=w185, index (row)=w184, index (col)=w183) -> (element=w182:sgl)
                n43 = call "Blend Overlay Color with Background.vi"("Overlay Color Value"=w176, "Image Scale Factor"=w175, "Blend Overlay with Background"=w179, "error in (no error)"=w174, "Image Display Range"=w177, "Image Color Array"=w178, "Pixel Value"=w182) -> ("error out"=w180:errorcluster, "Scaled/Blended Overlay Color Value"=w181:T4)  [unwired: 3 in]
                n44 = call "IMAQ ColorValueToInteger"("error in (no error)"=w180, "Color Value"=w181) -> ("error out"=w186:errorcluster, "U32 value"=w187:u32)  [unwired: 3 in, 2 out]
              }
            }
          }
          frame True {
            # "NaN"
          }
        }
      }
      n45 = Merge Errors(w121) -> (w120:errorcluster)
    }
    n46 = Merge Errors(w76) -> (w74:errorcluster)
    n47 = call "IMAQ Overlay Bitmap"("Group"="Decay Fit Parameter Color Map Overlay", "error in (no error)"=w74, "Bitmap"=w75, "Image"=w69) -> ("error out"=w78:errorcluster, "Image Out"=w115:T5)  [unwired: 6 in]
    n48 = in-place-dvr #1() -> (→"AlliGator IV DVR out":refnum<data-value>, w42:errorcluster)  [unwired: 1 in]
  }
  n49 = call "High Resolution Timing.vi"("relative seconds (NaN)"=w20, "Error In"=w42) -> ("relative seconds"=w18:dbl, "elapsed (relative) seconds"=→"Overlay Compute (s)":dbl, "Error Out"=w21:errorcluster)  [unwired: 15 in]
  n50 = Merge Errors(w21, w16) -> (w17:errorcluster)
  n51 = call "IMAQ Clear Overlay"("error in (no error)"=w17, "Image"=w55) -> ("error out"=w52:errorcluster, "Image Out"=w59:T5)  [unwired: 8 in]
  n52 = Add Array Elements(numeric array=w60) -> (sum=→"# Overlay Pixels":i32)
  n53 = call <vilib>:"Clear Errors.vi"("error in (no error)"=w52, "specific error code to clear (0: all)"=w51) -> ("error out"=w49:errorcluster)  [unwired: 4 in, 1 out]
  n54 = call "High Resolution Timing.vi"("relative seconds (NaN)"=w18, "Error In"=w49) -> ("relative seconds"=w46:dbl, "elapsed (relative) seconds"=→"Overlay Erase (s)":dbl, "Error Out"=w44:errorcluster)  [unwired: 15 in]
  n55 = call "IMAQ Copy Overlay"("error in (no error)"=w44, "Image Dst"=w59, "Image Src"=w41) -> ("error out"=w47:errorcluster, "Image Dst Out"=w58:T5)  [unwired: 7 in]
  n56 = call "High Resolution Timing.vi"("relative seconds (NaN)"=w46, "Error In"=w47) -> ("elapsed (relative) seconds"=→"Overlay Copy (s)":dbl, "Error Out"=w40:errorcluster)  [unwired: 15 in, 1 out]
  n57 = property class="ImageControl"(reference=w61, error in=w40, "Value"=w58) -> (error out=→"Error Out":errorcluster)  [unwired: 1 out]
  n58 = call "Tiny Clear Error.vi"("Error In"=w40) -> ("no Error Out"=w27:errorcluster)  [unwired: 8 in]
  n59 = call "IMAQ Dispose"("Image"=w41, "error in (no error)"=w27) -> ("error out"=w39:errorcluster)  [unwired: 4 in]
  n60 = call <vilib>:"Clear Errors.vi"("error in (no error)"=w39) -> ()  [unwired: 5 in, 2 out]
